vi "Drive Relative.vi"(6 "Distance From Target":dbl, 7 "Encoder Direction":bool, 8 "Encoder Reduction Factor":dbl, 9 "Angle Reduction Factor":dbl, 10 "Angle":dbl, 11 "Angle Direction":bool) -> (2 "Right Power":dbl, 3 "Left Power":dbl)   [LabVIEW 2016]
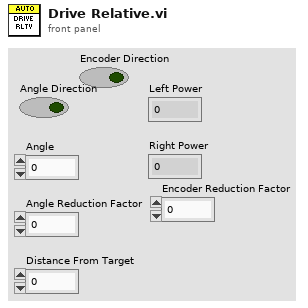
[diagram p1: front panel]
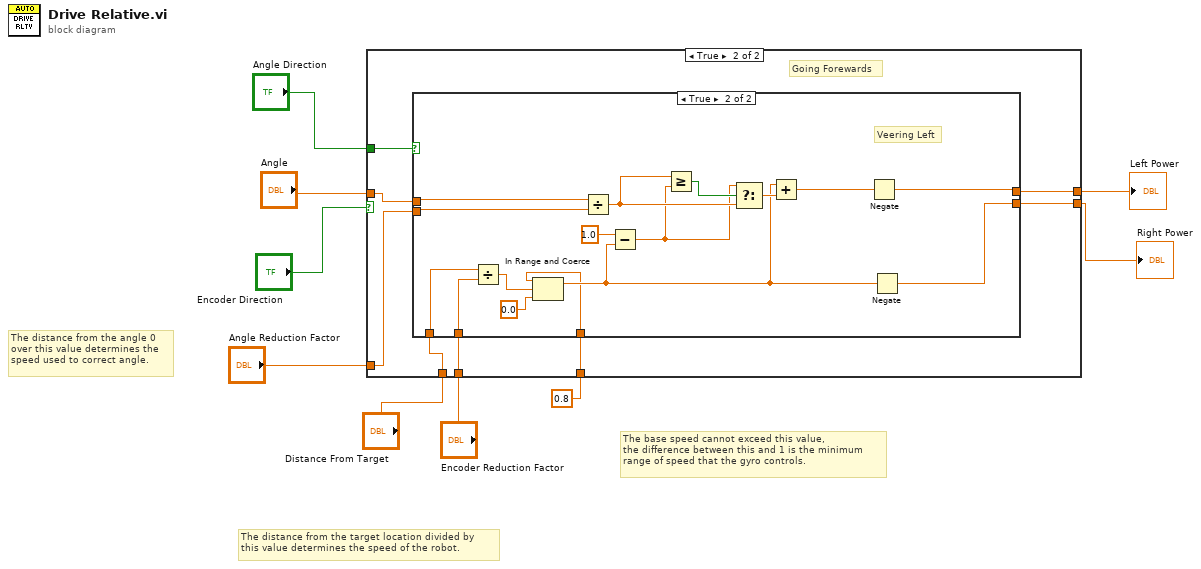
[diagram p0: block diagram]
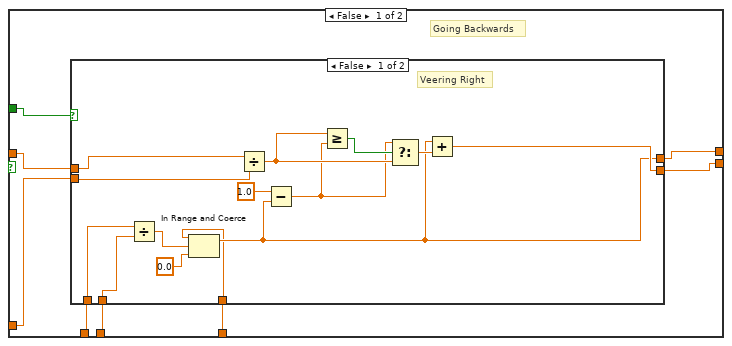
[diagram p2: hidden frame]
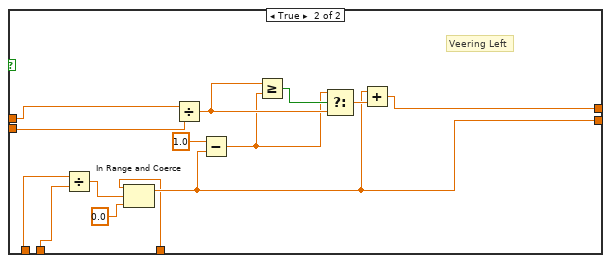
[diagram p3: hidden frame]
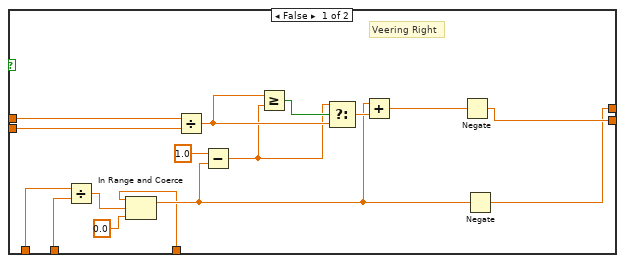
[diagram p4: hidden frame]
diagram:
  # "The distance from the angle 0\nover this value determines the \nspeed used to correct angle."
  # "The base speed cannot exceed this value,\nthe difference between this and 1 is the minimum\nrange of speed that the gyro controls."
  # "The distance from the target location divided by \nthis value determines the speed of the robot."
  n1 = case shown="True" "Encoder Direction" {
    tunnel: "Distance From Target" -> [w11 w53]
    tunnel: [w12 w52] -> w8
    tunnel: [w13 w51] -> w7
    tunnel: "Angle Reduction Factor" -> [w15 w50]
    tunnel: "Angle" -> [w16 w49]
    tunnel: "Angle Direction" -> [w14 w48]
    tunnel: "Encoder Reduction Factor" -> [w17 w47]
    tunnel: 0.8 ("upper limit") -> [w10 w46]
    frame False {
      # "Going Backwards"
      n2 = case shown="False" w14 {
        tunnel: [w19 w34] -> w13
        tunnel: [w20 w33] -> w12
        tunnel: w16 -> [w24 w37]
        tunnel: w15 -> [w23 w38]
        tunnel: w17 -> [w22 w36]
        tunnel: w11 -> [w21 w35]
        tunnel: w10 -> [w18 w32]
        frame False {
          # "Veering Right"
          n3 = Divide(x=w21, y=w22) -> (x/y=w27:dbl)
          n4 = In Range and Coerce(upper limit=w18, x=w27, lower limit=0.0) -> (coerced(x)=w19:dbl)  [unwired: 1 out]
          n5 = Divide(x=w24, y=w23) -> (x/y=w29:dbl)
          n6 = Subtract(x=1.0, y=w19) -> (x-y=w25:dbl)
          n7 = Greater Or Equal?(x=w29, y=w25) -> (x >= y?=w31:bool)
          n8 = Select(t=w25, s=w31, f=w29) -> (s? t:f=w30:dbl)
          n9 = Add(x=w19, y=w30) -> (x+y=w20:dbl)
        }
        frame True {
          # "Veering Left"
          n10 = Divide(x=w35, y=w36) -> (x/y=w41:dbl)
          n11 = In Range and Coerce(upper limit=w32, x=w41, lower limit=0.0) -> (coerced(x)=w33:dbl)  [unwired: 1 out]
          n12 = Divide(x=w37, y=w38) -> (x/y=w43:dbl)
          n13 = Subtract(x=1.0, y=w33) -> (x-y=w39:dbl)
          n14 = Greater Or Equal?(x=w43, y=w39) -> (x >= y?=w45:bool)
          n15 = Select(t=w39, s=w45, f=w43) -> (s? t:f=w44:dbl)
          n16 = Add(x=w33, y=w44) -> (x+y=w34:dbl)
        }
      }
    }
    frame True {
      # "Going Forewards"
      n17 = case shown="True" w48 {
        tunnel: [w55 w72] -> w51
        tunnel: [w57 w71] -> w52
        tunnel: w49 -> [w66 w76]
        tunnel: w50 -> [w65 w75]
        tunnel: w53 -> [w62 w74]
        tunnel: w47 -> [w63 w73]
        tunnel: w46 -> [w54 w70]
        frame False {
          # "Veering Right"
          n18 = Divide(x=w62, y=w63) -> (x/y=w61:dbl)
          n19 = In Range and Coerce(upper limit=w54, x=w61, lower limit=0.0) -> (coerced(x)=w56:dbl)  [unwired: 1 out]
          n20 = Divide(x=w66, y=w65) -> (x/y=w67:dbl)
          n21 = Subtract(x=1.0, y=w56) -> (x-y=w59:dbl)
          n22 = Greater Or Equal?(x=w67, y=w59) -> (x >= y?=w69:bool)
          n23 = Select(t=w59, s=w69, f=w67) -> (s? t:f=w68:dbl)
          n24 = Add(x=w56, y=w68) -> (x+y=w58:dbl)
          n25 = Negate(x=w58) -> (-x=w57:dbl)
          n26 = Negate(x=w56) -> (-x=w55:dbl)
        }
        frame True {
          # "Veering Left"
          n27 = Divide(x=w74, y=w73) -> (x/y=w81:dbl)
          n28 = In Range and Coerce(upper limit=w70, x=w81, lower limit=0.0) -> (coerced(x)=w77:dbl)  [unwired: 1 out]
          n29 = Divide(x=w76, y=w75) -> (x/y=w83:dbl)
          n30 = Subtract(x=1.0, y=w77) -> (x-y=w79:dbl)
          n31 = Greater Or Equal?(x=w83, y=w79) -> (x >= y?=w85:bool)
          n32 = Select(t=w79, s=w85, f=w83) -> (s? t:f=w84:dbl)
          n33 = Add(x=w77, y=w84) -> (x+y=w78:dbl)
          n34 = Negate(x=w78) -> (-x=w72:dbl)
          n35 = Negate(x=w77) -> (-x=w71:dbl)
        }
      }
    }
  }
  "Right Power" <- w8
  "Left Power" <- w7
